vi "校准画面.vi"() -> ()   [LabVIEW 2016, in "斯坦道原位多参数.lvlib"]
panel:
  in  "第三点取值":bool
  in  "第二点取值":bool
  in  "第一点取值":bool
  out "实时信号值":sgl caption="信号值："
  out "实时检测值":sgl caption="检测值："
  in  "校准记录写入":bool
  in  "校准记录读取":bool
  in  "第三点信号值":sgl
  in  "第三点检测值":sgl
  in  "第三点标准值":sgl caption="第三点："
  in  "第二点信号值":sgl
  in  "第二点检测值":sgl
  in  "第二点标准值":sgl caption="第二点："
  in  "第一点信号值":sgl
  in  "第一点检测值":sgl
  in  "第一点标准值":sgl caption="第一点："
  out "传感器温度":sgl caption="传感器温度："
  in  "校准类型":u16(ring) caption="校准类型：" items=["单点校准"=1, "两点校准"=2, "三点校准"=3]
  out "校准时间":timestamp caption="校准时间：" format="%<%x %X>T"
  out "SN":string caption="探头序列号："
  in  "校准探头":u16(ring)=9 caption="校准探头：" items=["水温"=9, "pH值"=10, "溶解氧"=11, "电导率"=12, "浊度"=13, "叶绿素a"=14, "藻密度"=15, "氧化还原电位"=17, "溶解氧%"=18, "盐度"=19]
  # "探头校准"
  # "标准值"
  # "检测值"
  # "信号值"
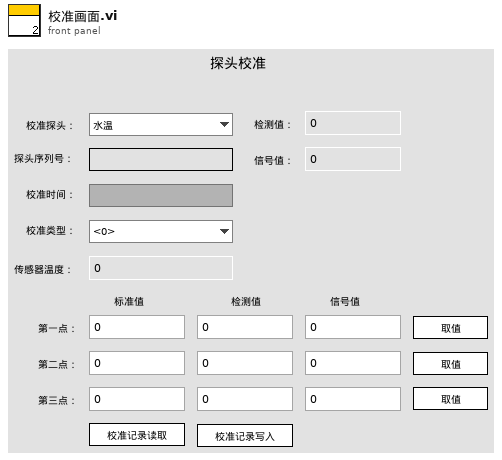
[diagram p1: front panel]
types:
  T1 = cluster{"SN":string, "时间标识":timestamp, "校准类型":u16, "传感器温度":sgl, "第一点标准值":sgl, "第二点标准值":sgl, "第三点标准值":sgl, "第一点检测值":sgl, "第二点检测值":sgl, "第三点检测值":sgl, "第一点原始值":sgl, "第二点原始值":sgl, "第三点原始值":sgl}
  T2 = cluster{"因子编码":string, "单位":string, "标样参考值":sgl, "水样数据时间":timestamp, "水样实测值":sgl, "水样数据标识":string, "K":sgl, "B":sgl, "T":sgl, "H":sgl, "水深":sgl, "探头温度":sgl, "信号值":sgl}
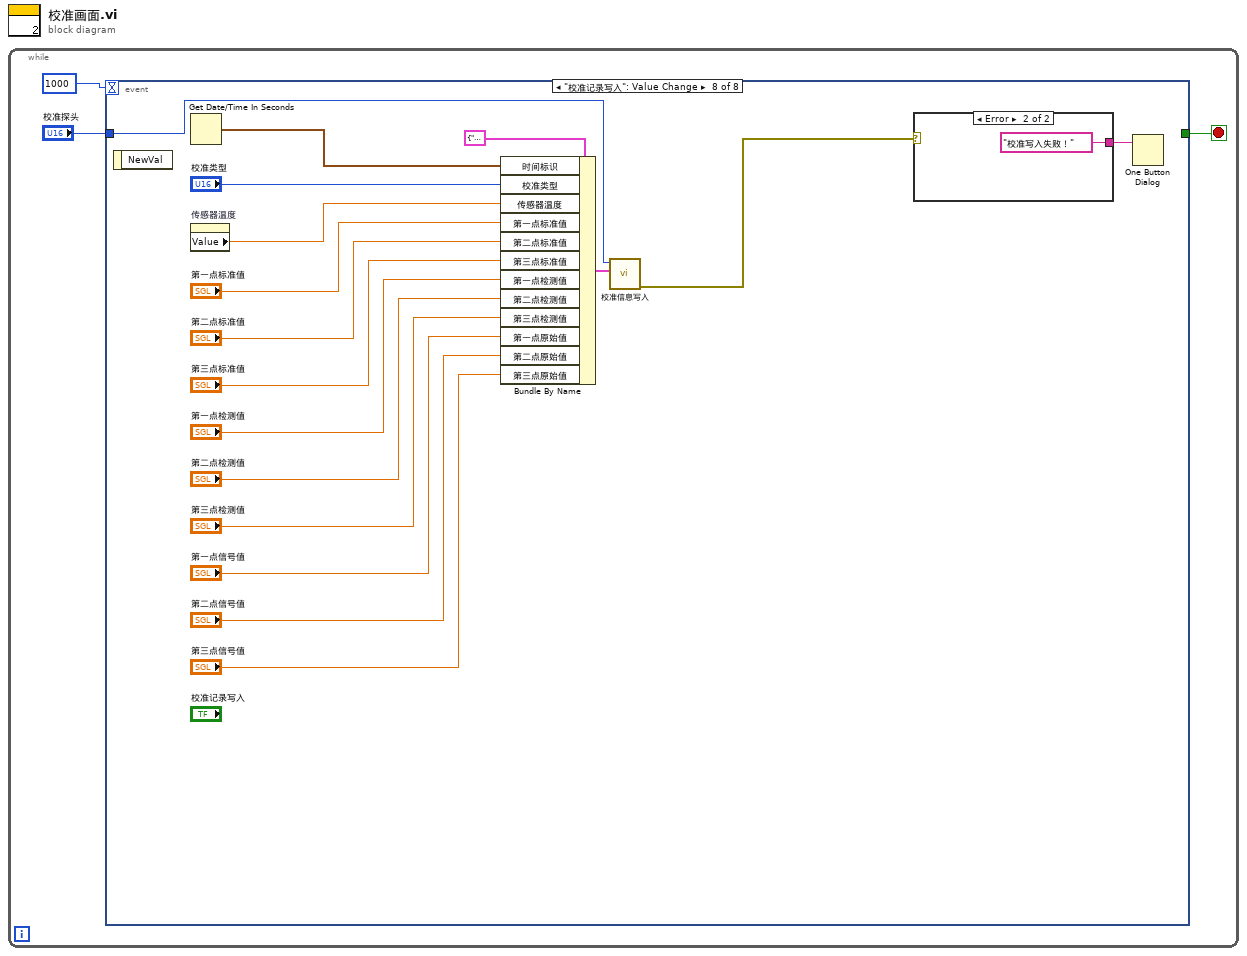
[diagram p0: block diagram]
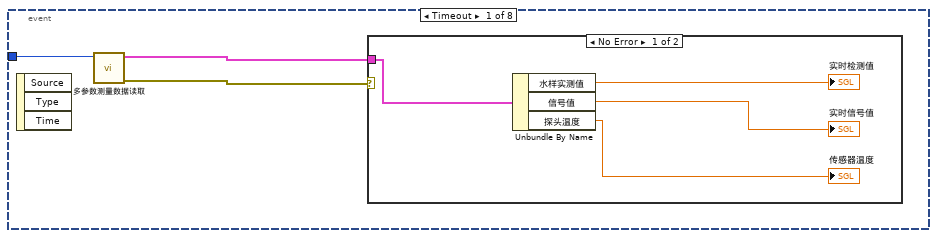
[diagram p2: hidden frame]
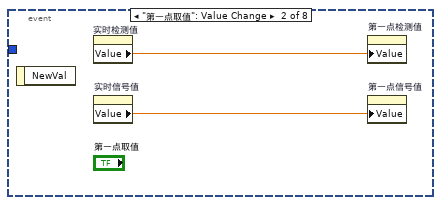
[diagram p4: hidden frame]
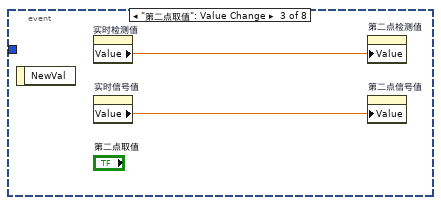
[diagram p5: hidden frame]
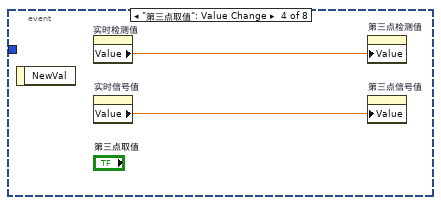
[diagram p6: hidden frame]
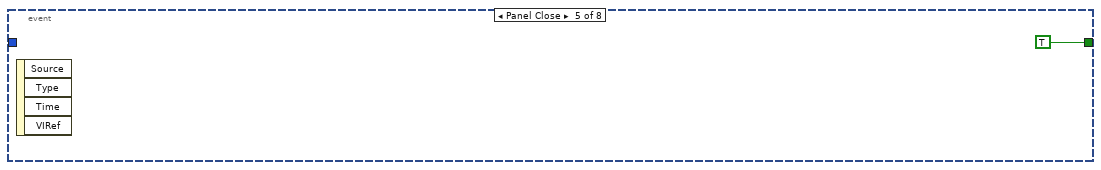
[diagram p7: hidden frame]
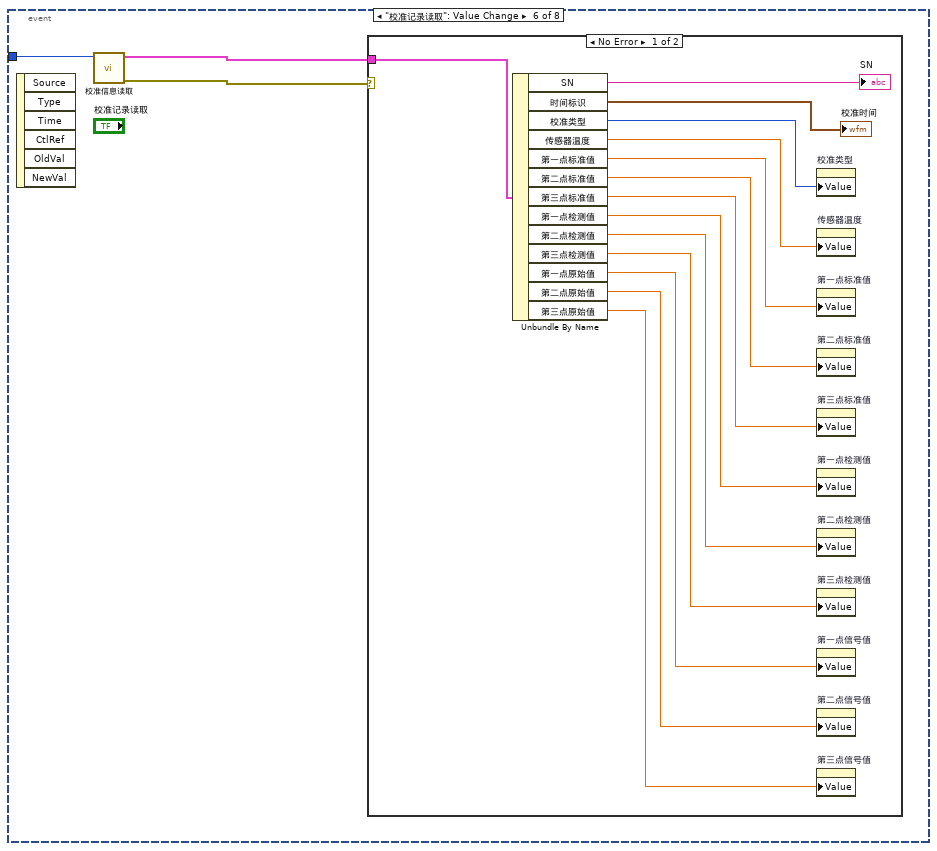
[diagram p8: hidden frame]
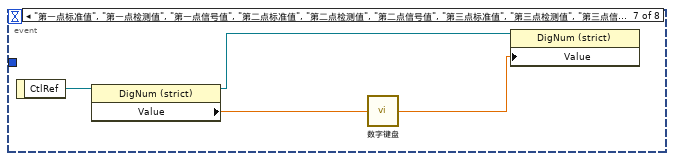
[diagram p10: hidden frame]
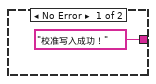
[diagram p11: hidden frame]
diagram:
  n1 = while {
    stop <- w3 stop-if-true
    n2 = event shown="[7] \"校准记录写入\": Value Change" {
      selector: _ -> [_ _ _ _ _ _ _ _]
      dyn-events: _ -> [_ _ _ _ _ _ _ _]
      timeout: 1000 -> [_ _ _ _ _ _ _ _]
      tunnel: [_ _ _ _ TRUE _ _ _] -> w3
      tunnel: "校准探头" -> [w6 _ _ _ _ w18 _ w55]
      event Timeout {
        n3 = event-data() -> ()  [unwired: 1 in, 3 out]
        n4 = call "多参数测量数据读取.vi"("探头选择"=w6) -> ("error out"=w4:errorcluster, "测量数据块"=w5:T2)  [unwired: 8 in, 1 out]
        n5 = case shown="No Error" w4 {
          tunnel: w5 -> [w10 _]
          frame No Error {
            n6 = Unbundle By Name(w10) -> ("水样实测值"=→"实时检测值":sgl, "信号值"=→"实时信号值":sgl, "探头温度"=→"传感器温度":sgl)
          }
          frame Error {
          }
        }
      }
      event "第一点取值": Value Change {
        n7 = event-data() -> ()  [unwired: 1 in, 1 out]
        n8 = property on="实时检测值" class="DigNum (strict)"() -> ("Value"=w12:sgl)  [unwired: 2 in, 2 out]
        n9 = property on="实时信号值" class="DigNum (strict)"() -> ("Value"=w11:sgl)  [unwired: 2 in, 2 out]
        n10 = property on="第一点检测值" class="DigNum (strict)"("Value"=w12) -> ()  [unwired: 2 in, 2 out]
        n11 = property on="第一点信号值" class="DigNum (strict)"("Value"=w11) -> ()  [unwired: 2 in, 2 out]
      }
      event "第二点取值": Value Change {
        n12 = event-data() -> ()  [unwired: 1 in, 1 out]
        n13 = property on="实时检测值" class="DigNum (strict)"() -> ("Value"=w14:sgl)  [unwired: 2 in, 2 out]
        n14 = property on="实时信号值" class="DigNum (strict)"() -> ("Value"=w13:sgl)  [unwired: 2 in, 2 out]
        n15 = property on="第二点检测值" class="DigNum (strict)"("Value"=w14) -> ()  [unwired: 2 in, 2 out]
        n16 = property on="第二点信号值" class="DigNum (strict)"("Value"=w13) -> ()  [unwired: 2 in, 2 out]
      }
      event "第三点取值": Value Change {
        n17 = event-data() -> ()  [unwired: 1 in, 1 out]
        n18 = property on="实时检测值" class="DigNum (strict)"() -> ("Value"=w16:sgl)  [unwired: 2 in, 2 out]
        n19 = property on="实时信号值" class="DigNum (strict)"() -> ("Value"=w15:sgl)  [unwired: 2 in, 2 out]
        n20 = property on="第三点检测值" class="DigNum (strict)"("Value"=w16) -> ()  [unwired: 2 in, 2 out]
        n21 = property on="第三点信号值" class="DigNum (strict)"("Value"=w15) -> ()  [unwired: 2 in, 2 out]
      }
      event Panel Close {
        n22 = event-data() -> ()  [unwired: 1 in, 4 out]
      }
      event "校准记录读取": Value Change {
        n23 = event-data() -> ()  [unwired: 1 in, 6 out]
        n24 = call "校准信息读取.vi"("Slave ID"=w18) -> ("error out"=w19:errorcluster, "校准信息读取"=w20:T1)  [unwired: 9 in]
        n25 = case shown="No Error" w19 {
          tunnel: w20 -> [w34 _]
          frame No Error {
            n26 = Unbundle By Name(w34) -> ("SN"=→"SN":string, "时间标识"=→"校准时间":timestamp, "校准类型"=w31:u16, "传感器温度"=w30:sgl, "第一点标准值"=w29:sgl, "第二点标准值"=w28:sgl, "第三点标准值"=w27:sgl, "第一点检测值"=w26:sgl, "第二点检测值"=w25:sgl, "第三点检测值"=w24:sgl, "第一点原始值"=w23:sgl, "第二点原始值"=w22:sgl, "第三点原始值"=w21:sgl)
            n27 = property on="校准类型" class="Ring (strict)"("Value"=w31) -> ()  [unwired: 2 in, 2 out]
            n28 = property on="传感器温度" class="DigNum (strict)"("Value"=w30) -> ()  [unwired: 2 in, 2 out]
            n29 = property on="第一点标准值" class="DigNum (strict)"("Value"=w29) -> ()  [unwired: 2 in, 2 out]
            n30 = property on="第二点标准值" class="DigNum (strict)"("Value"=w28) -> ()  [unwired: 2 in, 2 out]
            n31 = property on="第三点标准值" class="DigNum (strict)"("Value"=w27) -> ()  [unwired: 2 in, 2 out]
            n32 = property on="第一点检测值" class="DigNum (strict)"("Value"=w26) -> ()  [unwired: 2 in, 2 out]
            n33 = property on="第二点检测值" class="DigNum (strict)"("Value"=w25) -> ()  [unwired: 2 in, 2 out]
            n34 = property on="第三点检测值" class="DigNum (strict)"("Value"=w24) -> ()  [unwired: 2 in, 2 out]
            n35 = property on="第一点信号值" class="DigNum (strict)"("Value"=w23) -> ()  [unwired: 2 in, 2 out]
            n36 = property on="第二点信号值" class="DigNum (strict)"("Value"=w22) -> ()  [unwired: 2 in, 2 out]
            n37 = property on="第三点信号值" class="DigNum (strict)"("Value"=w21) -> ()  [unwired: 2 in, 2 out]
          }
          frame Error {
          }
        }
      }
      event "第一点标准值", "第一点检测值", "第一点信号值", "第二点标准值", "第二点检测值", "第二点信号值", "第三点标准值", "第三点检测值", "第三点信号值": Mouse Down {
        n38 = event-data() -> ("CtlRef"=w38:refnum<vi>)  [unwired: 1 in]
        n39 = property class="DigNum (strict)"(reference=w38) -> (reference out=w35:refnum<vi>, "Value"=w37:sgl)  [unwired: 1 in, 1 out]
        n40 = call "数字键盘.vi"("OldNumber"=w37) -> ("NewNumber"=w36:dbl)
        n41 = property class="DigNum (strict)"(reference=w35, "Value"=w36) -> ()  [unwired: 1 in, 2 out]
      }
      event "校准记录写入": Value Change {
        n42 = event-data() -> ()  [unwired: 1 in, 1 out]
        n43 = Get Date/Time In Seconds() -> (seconds since 1Jan1904=w52:timestamp)
        n44 = property on="传感器温度" class="DigNum (strict)"() -> ("Value"=w50:sgl)  [unwired: 2 in, 2 out]
        n45 = Bundle By Name(cluster=T1 {"SN"="", "时间标识"=timestamp(0 s since 1904-01-01), "校准类型"=0, "传感器温度"=0.0, "第一点标准值"=0.0, "第二点标准值"=0.0, "第三点标准值"=0.0, "第一点检测值"=0.0, "第二点检测值"=0.0, "第三点检测值"=0.0, "第一点原始值"=0.0, "第二点原始值"=0.0, "第三点原始值"=0.0} ("校准信息读取"), "时间标识"=w52, "校准类型"="校准类型", "传感器温度"=w50, "第一点标准值"="第一点标准值", "第二点标准值"="第二点标准值", "第三点标准值"="第三点标准值", "第一点检测值"="第一点检测值", "第二点检测值"="第二点检测值", "第三点检测值"="第三点检测值", "第一点原始值"="第一点信号值", "第二点原始值"="第二点信号值", "第三点原始值"="第三点信号值") -> (w53:T1)
        n46 = call "校准信息写入.vi"("校准信息读取"=w53, "Slave ID"=w55) -> ("error out"=w40:errorcluster)  [unwired: 9 in]
        n47 = case shown="Error" w40 {
          tunnel: ["校准写入成功！" "校准写入失败！"] -> w39
          frame No Error {
          }
          frame Error {
          }
        }
        n48 = One Button Dialog(message=w39) -> ()  [unwired: 1 in, 1 out]
      }
    }
  }
